vi "DiffDrvAccelLimit_New.vi"(6 "MaxAngularAcceleration":dbl, 8 "MaxLinearAcceleration":dbl, 9 "MinLinearAcceleration":dbl, 10 "TrackWidth":dbl, 11 "LINEARSYSTEM":T1) -> (0 "Error":bool, 3 "outDiffDriveAccelLimit":T3)   [LabVIEW 2019, in "Trajectory_Library.lvlib"]
doc: "Constructs a DifferentialDriveAccelerationLimiter data cluster.\n \nInputs:\n - system -- The differential drive dynamics.\n - trackwidth -- The trackwidth.\n - minLinearAccel -- The minimum (most negative) linear acceleration in meters per second squared.\n - maxLinearAccel -- The maximum (most positive) linear acceleration in meters per second squared.\n\nOutputs:\n - DiffDriveAccelLimit -- Created data cluster\n - Error -- True if an error occured. (Min Accel limit is > than Max Accel Limit )"
uses:
  Trajectory_Library.lvlib
  TypeDef/DIFF_DRIVE_ACCEL_LIMIT.ctl
  TypeDef/LINEAR_SYSTEM.ctl
  <vilib>/Analysis/Matrix/Datatypes/RealMatrix.ctl
  <vilib>/Analysis/Matrix/NI_Matrix.lvlib
panel:
  # "<States,States>"
  # "<States,Inputs>"
  # "<Outputs,States>"
  # "<Outputs,Inputs>"
  # "<States,States>"
  # "<States,Inputs>"
  # "<Outputs,States>"
  # "<Outputs,Inputs>"
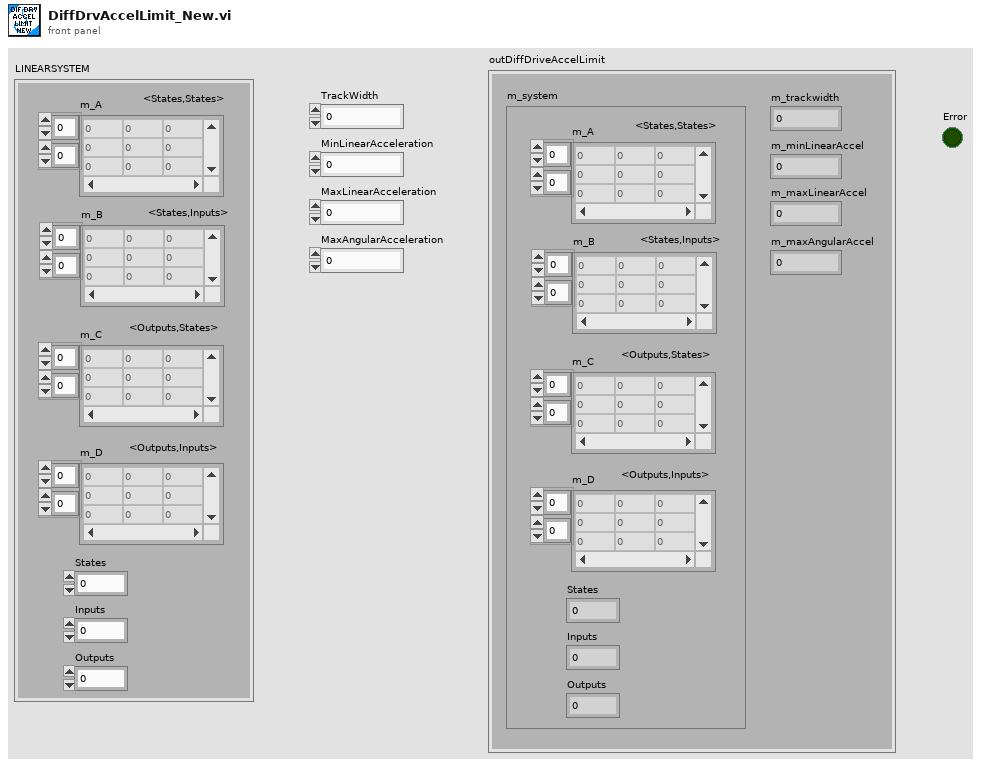
[diagram p1: front panel]
types:
  T1 = typedef "Trajectory_Library.lvlib/LINEAR_SYSTEM.ctl" = cluster{"m_A":T2, "m_B":T2, "m_C":T2, "m_D":T2, "States":i32, "Inputs":i32, "Outputs":i32}
  T2 = typedef "NI_Matrix.lvlib/RealMatrix.ctl" = dbl[][]
  T3 = typedef "Trajectory_Library.lvlib/DIFF_DRIVE_ACCEL_LIMIT.ctl" = cluster{"m_system":T1, "m_trackwidth":dbl, "m_maxLinearAccel":dbl, "m_maxAngularAccel":dbl, "m_minLinearAccel":dbl}
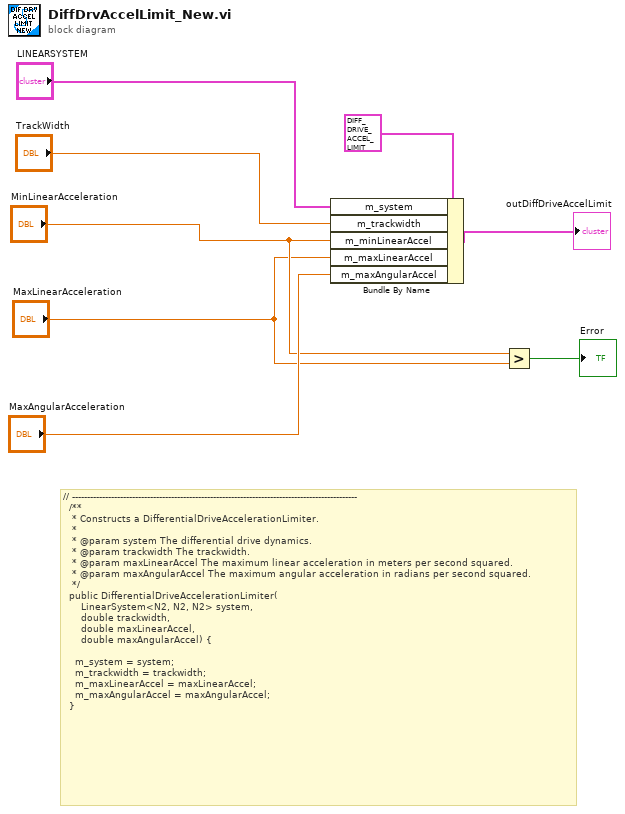
[diagram p0: block diagram]
diagram:
  # "// -----------------------------------------------------------------------------------------------\n  /**\n   * Constructs a DifferentialDriveAccelerationLimiter.\n   *\n   * @param system The differential drive dynamics.\n   * @param trackwidth The trackwidth.\n   * @param maxLinearAccel The maximum linear acceleration in meters per second squared.\n   * @param maxAngularAccel The maximum angular acceleration in radians per second squared.\n   */\n  public DifferentialDriveAccelerationLimiter(\n      LinearSystem<N2, N2, N2> system,\n      double trackwidth,\n      double maxLinearAccel,\n      double maxAngularAccel) {\n\n    m_system = system;\n    m_trackwidth = trackwidth;\n    m_maxLinearAccel = maxLinearAccel;\n    m_maxAngularAccel = maxAngularAccel;\n  }"
  n1 = Bundle By Name(cluster=T3 {"m_system"={"m_A"=[], "m_B"=[], "m_C"=[], "m_D"=[], "States"=0, "Inputs"=0, "Outputs"=0}, "m_trackwidth"=0.0, "m_maxLinearAccel"=0.0, "m_maxAngularAccel"=0.0, "m_minLinearAccel"=0.0} ("DIFF_DRIVE_ACCEL_LIMIT"), "m_system"="LINEARSYSTEM", "m_trackwidth"="TrackWidth", "m_minLinearAccel"="MinLinearAcceleration", "m_maxLinearAccel"="MaxLinearAcceleration", "m_maxAngularAccel"="MaxAngularAcceleration") -> (→"outDiffDriveAccelLimit":T3)
  n2 = Greater?(x="MinLinearAcceleration", y="MaxLinearAcceleration") -> (0:→"Error":bool)
